vi "DeviceStripSub1.vi"(10 "Individual Module Information Array":string[][](array[string])) -> (2 "Formatted Module Information":T1)   [LabVIEW 2016]
uses:
  Control/Control_ModuleArray.ctl
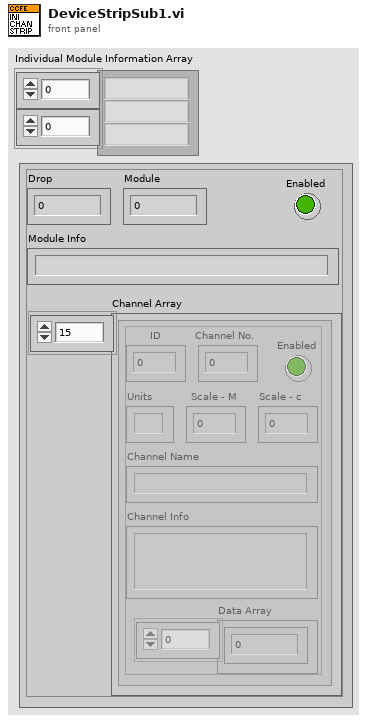
[diagram p1: front panel]
types:
  T1 = cluster{"Drop":i32, "Module":i32, "Module Info":string, "Enabled":bool, "Channel Array":cluster{"ID":i32, "Channel No.":i32, "Enabled":bool, "Channel Name":string, "Channel Info":string, "Units":string, "Scale - M":dbl, "Scale - c":dbl, "Data Array":dbl[]}[]}
  T2 = cluster{"ID":i32, "Channel No.":i32, "Enabled":bool, "Channel Name":string, "Channel Info":string, "Units":string, "Scale - M":dbl, "Scale - c":dbl, "Data Array":dbl[]}[]
  T3 = typedef "Control_ModuleArray.ctl" = cluster{"Drop":i32, "Module":i32, "Module Info":string, "Enabled":bool, "Channel Array":cluster{"ID":i32, "Channel No.":i32, "Enabled":bool, "Channel Name":string, "Channel Info":string, "Units":string, "Scale - M":dbl, "Scale - c":dbl, "Data Array":dbl[]}[]}[]
  T4 = cluster{"ID":i32, "Channel No.":i32, "Enabled":bool, "Channel Name":string, "Channel Info":string, "Units":string, "Scale - M":dbl, "Scale - c":dbl, "Data Array":dbl[]}
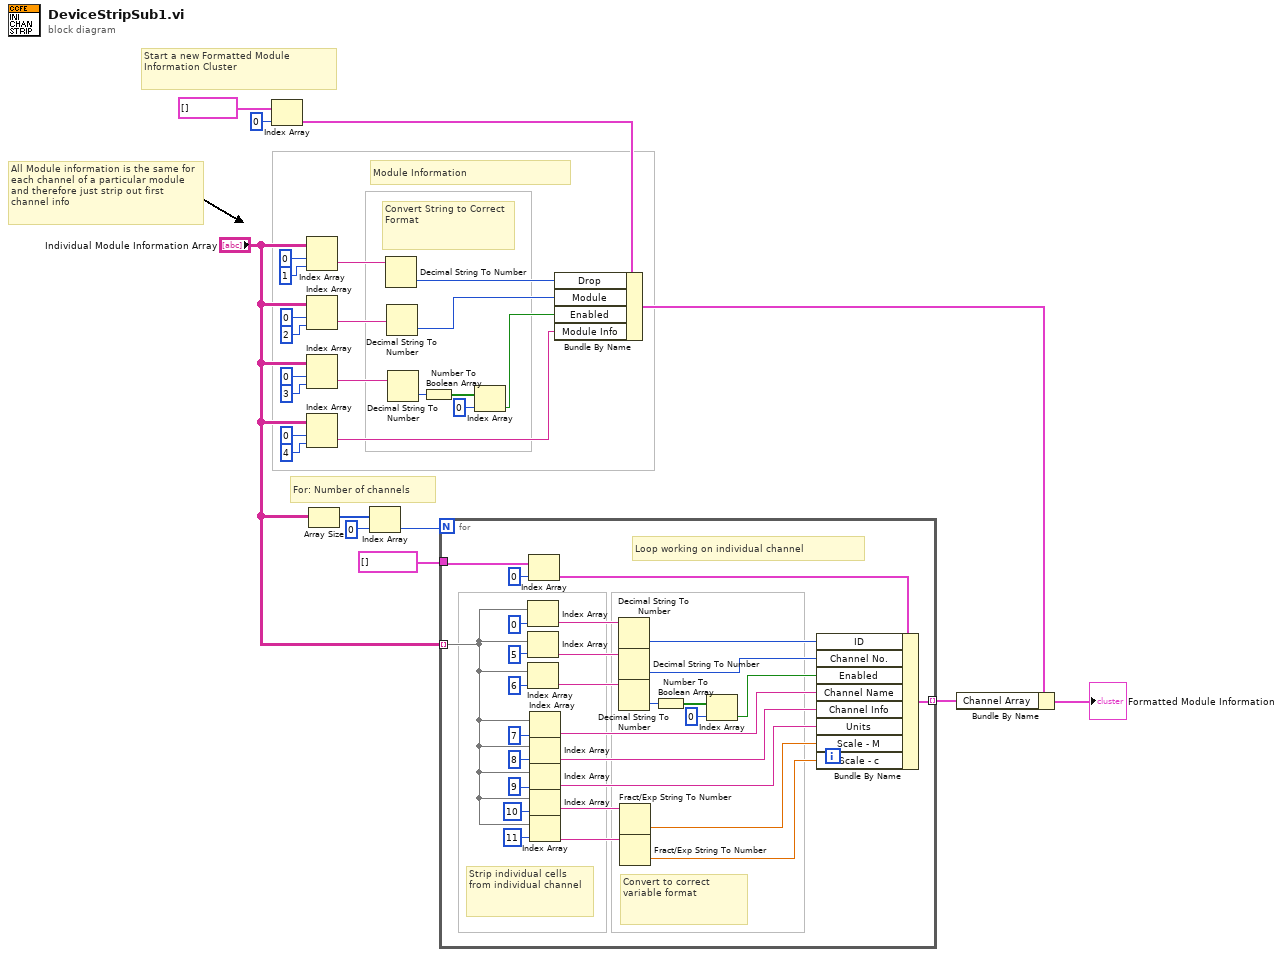
[diagram p0: block diagram]
diagram:
  # "Module Information"
  # "For: Number of channels"
  # "Convert String to Correct Format"
  # "Start a new Formatted Module Information Cluster"
  # "All Module information is the same for each channel of a particular module and therefore just strip out first channel info"
  n1 = Index Array(array=T3 [] ("Module Array"), index=0) -> (element=w8:T1)
  n2 = Index Array(array="Individual Module Information Array", index (row)=0 ("index"), index (col)=1 ("disabled index (col)")) -> (element=w9:string)
  n3 = Index Array(array="Individual Module Information Array", index (row)=0 ("index"), index (col)=2 ("disabled index (col)")) -> (element=w11:string)
  n4 = Index Array(array="Individual Module Information Array", index (row)=0 ("index"), index (col)=3 ("disabled index (col)")) -> (element=w17:string)
  n5 = Index Array(array="Individual Module Information Array", index (row)=0 ("index"), index (col)=4 ("disabled index (col)")) -> (element=w24:string)
  n6 = Array Size(array="Individual Module Information Array") -> (size(s)=w26:i32[])
  n7 = Index Array(array=w26, index=0) -> (element=w29:i32)
  n8 = Decimal String To Number(string=w9) -> (number=w10:i32)  [unwired: 2 in, 1 out]
  n9 = Decimal String To Number(string=w11) -> (number=w14:i32)  [unwired: 2 in, 1 out]
  n10 = Decimal String To Number(string=w17) -> (number=w18:i32)  [unwired: 2 in, 1 out]
  n11 = Number To Boolean Array(number=w18) -> (Boolean array=w20:bool[])
  n12 = for {
    N: w29 -> [_]
    tunnel: "Individual Module Information Array" -> [w34] mode=indexing
    tunnel: T2 [] ("Channel Array") -> [w33]
    tunnel: [w30] -> w28 mode=indexing
    # "Convert to correct variable format"
    # "Loop working on individual channel"
    # "Strip individual cells from individual channel"
    n13 = Index Array(array=w34, index=0) -> (element=w57:string)
    n14 = Index Array(array=w34, index=5) -> (element=w54:string)
    n15 = Index Array(array=w34, index=6) -> (element=w48:string)
    n16 = Index Array(array=w33, index=0) -> (element=w31:T4)
    n17 = Index Array(array=w34, index=7) -> (element=w44:string)
    n18 = Index Array(array=w34, index=8) -> (element=w43:string)
    n19 = Index Array(array=w34, index=9) -> (element=w41:string)
    n20 = Index Array(array=w34, index=10) -> (element=w38:string)
    n21 = Index Array(array=w34, index=11) -> (element=w36:string)
    n22 = Decimal String To Number(string=w57) -> (number=w56:i32)  [unwired: 2 in, 1 out]
    n23 = Decimal String To Number(string=w54) -> (number=w53:i32)  [unwired: 2 in, 1 out]
    n24 = Decimal String To Number(string=w48) -> (number=w50:i32)  [unwired: 2 in, 1 out]
    n25 = Fract/Exp String To Number(string=w38) -> (number=w37:dbl)  [unwired: 3 in, 1 out]
    n26 = Fract/Exp String To Number(string=w36) -> (number=w35:dbl)  [unwired: 3 in, 1 out]
    n27 = Number To Boolean Array(number=w50) -> (Boolean array=w52:bool[])
    n28 = Index Array(array=w52, index=0) -> (element=w47:bool)
    n29 = Bundle By Name(cluster=w31, "ID"=w56, "Channel No."=w53, "Enabled"=w47, "Channel Name"=w44, "Channel Info"=w43, "Units"=w41, "Scale - M"=w37, "Scale - c"=w35) -> (w30:T4)
  }
  n30 = Index Array(array=w20, index=0) -> (element=w21:bool)
  n31 = Bundle By Name(cluster=w8, "Drop"=w10, "Module"=w14, "Enabled"=w21, "Module Info"=w24) -> (w27:T1)
  n32 = Bundle By Name(cluster=w27, "Channel Array"=w28) -> (→"Formatted Module Information":T1)
